vi "Close.vi"(8 "error in (no error)":errorcluster, 11 "UndoObject in":refnum<class "UndoObject.lvclass">) -> (0 "error out":errorcluster)   [LabVIEW 2015, in "UndoLibrary.lvlib" / "UndoObject.lvclass"]
doc: "This VI destroys the references to store the values of the control."
uses:
  UndoObject.lvclass
  UndoObject.lvclass/UndoObject.ctl
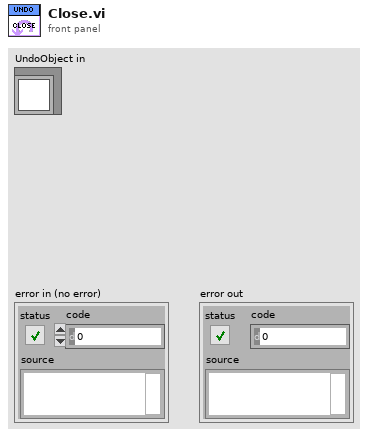
[diagram p1: front panel]
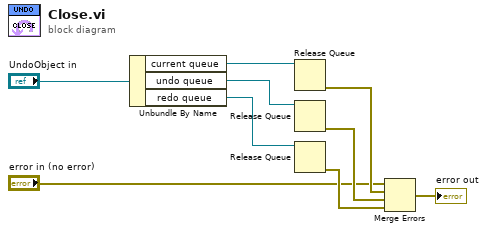
[diagram p0: block diagram]
diagram:
  n1 = Unbundle By Name("UndoObject in") -> ("current queue"=w3:refnum<queue>, "undo queue"=w4:refnum<queue>, "redo queue"=w5:refnum<queue>)
  n2 = Release Queue(queue=w3) -> (error out=w8:errorcluster)  [unwired: 2 in, 2 out]
  n3 = Release Queue(queue=w4) -> (error out=w7:errorcluster)  [unwired: 2 in, 2 out]
  n4 = Release Queue(queue=w5) -> (error out=w6:errorcluster)  [unwired: 2 in, 2 out]
  n5 = Merge Errors("error in (no error)", w8, w7, w6) -> (→"error out":errorcluster)
